vi "Write Iteration Index.vi"(8 "error in (no error)":errorcluster, 10 "Iteration Index":i32, 11 "Counter.lvclass":refnum<class "Counter.lvclass">) -> (0 "error out":errorcluster, 3 "Counter.lvclass":refnum<class "Counter.lvclass">)   [LabVIEW 2015, in "Counter.lvclass"]
uses:
  Counter.lvclass
  Counter.lvclass/Counter.ctl
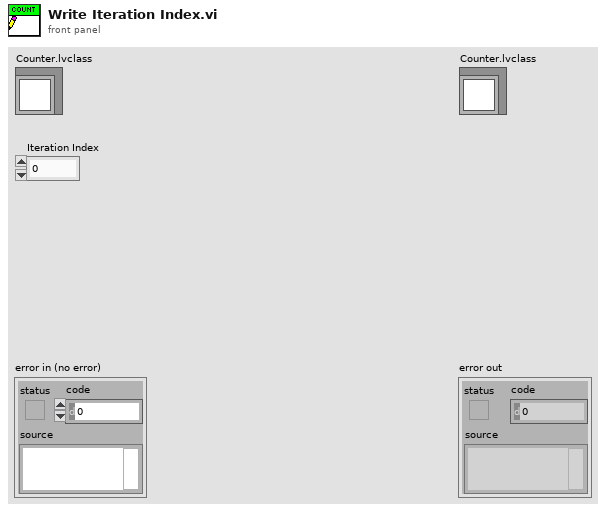
[diagram p1: front panel]
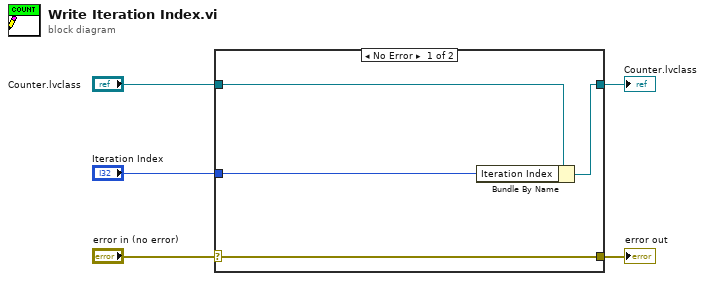
[diagram p0: block diagram]
diagram:
  n1 = case shown="No Error" "error in (no error)" {
    selector: "error in (no error)" -> [w9 w10]
    tunnel: [w9 w10] -> w4
    tunnel: [w7 w11] -> w2
    tunnel: "Counter.lvclass" -> [w8 w11]
    tunnel: "Iteration Index" -> [w6 _]
    frame No Error {
      n2 = Bundle By Name(cluster=w8, "Iteration Index"=w6) -> (w7:refnum<class "Counter.lvclass">)
    }
    frame Error {
    }
  }
  "error out" <- w4
  "Counter.lvclass" <- w2
